vi "Escape String for JSON.vi"(11 "string":string) -> (3 "quoted string":string)   [LabVIEW 2020, in "Multi Error Cluster.lvlib"]
doc: "Convert reserved JSON characters into \\ escaped character sequences. This allows a name to contain a /, '\", \\, or a control character."
uses:
  <vilib>/MultiError/TokenizeJSON/Multi Error Cluster.lvlib
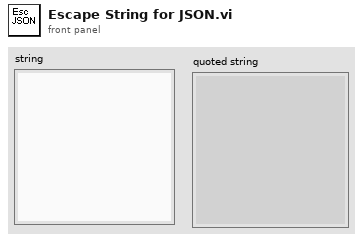
[diagram p1: front panel]
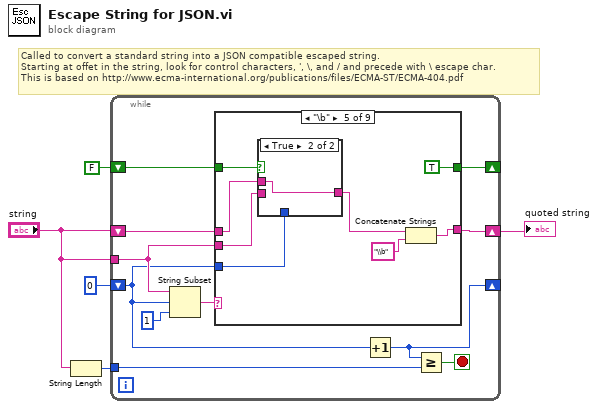
[diagram p0: block diagram]
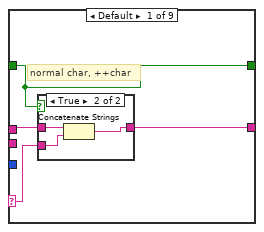
[diagram p2: hidden frame]
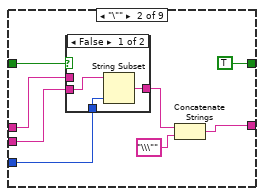
[diagram p4: hidden frame]
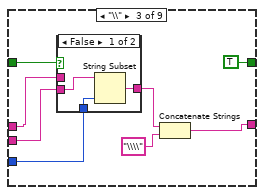
[diagram p6: hidden frame]
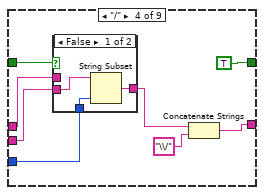
[diagram p8: hidden frame]
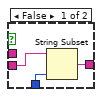
[diagram p10: hidden frame]
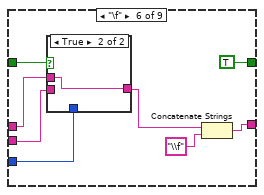
[diagram p11: hidden frame]
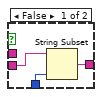
[diagram p12: hidden frame]
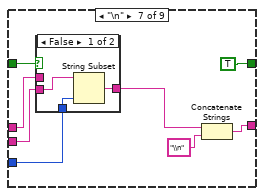
[diagram p13: hidden frame]
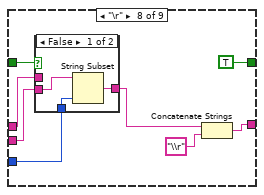
[diagram p15: hidden frame]
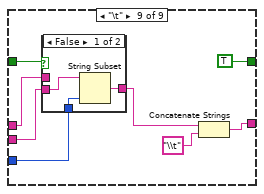
[diagram p17: hidden frame]
diagram:
  # "Called to convert a standard string into a JSON compatible escaped string.\nStarting at offet in the string, look for control characters, ', \\, and / and precede with \\ escape char.\nThis is based on http://www.ecma-international.org/publications/files/ECMA-ST/ECMA-404.pdf"
  n1 = String Length(string="string") -> (length=w5:i32)
  n2 = while {
    shift-right: [w10] -> w1
    shift-left: "string" -> [w11]
    shift-right: [w8] -> _
    shift-left: 0 ("offset") -> [w6]
    tunnel: w5 -> [w14]
    shift-right: [w9] -> _
    shift-left: FALSE -> [w12]
    tunnel: "string" -> [w7]
    stop <- w13 stop-if-true
    n3 = String Subset(string=w7, offset (0)=w6, length (rest)=1) -> (substring=w15:string)
    n4 = case shown="\"\\b\"" w15 {
      selector: w15 -> [w18 _ _ _ _ _ _ _ _]
      tunnel: w11 -> [w20 w28 w39 w52 w64 w77 w88 w100 w110]
      tunnel: w12 -> [w17 w29 w41 w53 w65 w75 w89 w101 w113]
      tunnel: [w19 w31 w43 w55 w67 w79 w91 w103 w115] -> w10
      tunnel: [w17 TRUE TRUE TRUE TRUE TRUE TRUE TRUE TRUE] -> w9
      tunnel: w7 -> [_ w27 w38 w51 w63 w76 w87 w99 w111]
      tunnel: w6 -> [_ w26 w37 w50 w62 w74 w86 w98 w112]
      frame Default {
        # "normal char, ++char"
        n5 = case shown="True" w17 {
          tunnel: w20 -> [w21 w24]
          tunnel: [w21 w22] -> w19
          tunnel: w18 -> [_ w23]
          frame False {
          }
          frame True {
            n6 = Concatenate Strings(w24, w23) -> (w22:string)
          }
        }
      }
      frame "\"" {
        n7 = case shown="False" w29 {
          tunnel: w28 -> [_ w36]
          tunnel: [w33 w36] -> w25
          tunnel: w27 -> [w35 _]
          tunnel: w26 -> [w34 _]
          frame False {
            n8 = String Subset(string=w35, length (rest)=w34) -> (substring=w33:string)  [unwired: 1 in]
          }
          frame True {
          }
        }
        n9 = Concatenate Strings(w25, "\\\"") -> (w31:string)
      }
      frame "\\" {
        n10 = case shown="False" w41 {
          tunnel: w39 -> [_ w48]
          tunnel: [w46 w48] -> w40
          tunnel: w37 -> [w47 _]
          tunnel: w38 -> [w45 _]
          frame False {
            n11 = String Subset(string=w45, length (rest)=w47) -> (substring=w46:string)  [unwired: 1 in]
          }
          frame True {
          }
        }
        n12 = Concatenate Strings(w40, "\\\\") -> (w43:string)
      }
      frame "/" {
        n13 = case shown="False" w53 {
          tunnel: w52 -> [_ w60]
          tunnel: [w57 w60] -> w49
          tunnel: w51 -> [w59 _]
          tunnel: w50 -> [w58 _]
          frame False {
            n14 = String Subset(string=w59, length (rest)=w58) -> (substring=w57:string)  [unwired: 1 in]
          }
          frame True {
          }
        }
        n15 = Concatenate Strings(w49, "\\/") -> (w55:string)
      }
      frame "\b" {
        n16 = case shown="True" w65 {
          tunnel: [w69 w72] -> w61
          tunnel: w63 -> [w71 _]
          tunnel: w62 -> [w70 _]
          tunnel: w64 -> [_ w72]
          frame False {
            n17 = String Subset(string=w71, length (rest)=w70) -> (substring=w69:string)  [unwired: 1 in]
          }
          frame True {
          }
        }
        n18 = Concatenate Strings(w61, "\\b") -> (w67:string)
      }
      frame "\f" {
        n19 = case shown="True" w75 {
          tunnel: [w81 w84] -> w73
          tunnel: w76 -> [w83 _]
          tunnel: w74 -> [w82 _]
          tunnel: w77 -> [_ w84]
          frame False {
            n20 = String Subset(string=w83, length (rest)=w82) -> (substring=w81:string)  [unwired: 1 in]
          }
          frame True {
          }
        }
        n21 = Concatenate Strings(w73, "\\f") -> (w79:string)
      }
      frame "\n" {
        n22 = case shown="False" w89 {
          tunnel: w88 -> [_ w96]
          tunnel: [w93 w96] -> w85
          tunnel: w87 -> [w95 _]
          tunnel: w86 -> [w94 _]
          frame False {
            n23 = String Subset(string=w95, length (rest)=w94) -> (substring=w93:string)  [unwired: 1 in]
          }
          frame True {
          }
        }
        n24 = Concatenate Strings(w85, "\\n") -> (w91:string)
      }
      frame "\r" {
        n25 = case shown="False" w101 {
          tunnel: w100 -> [_ w108]
          tunnel: [w105 w108] -> w97
          tunnel: w99 -> [w107 _]
          tunnel: w98 -> [w106 _]
          frame False {
            n26 = String Subset(string=w107, length (rest)=w106) -> (substring=w105:string)  [unwired: 1 in]
          }
          frame True {
          }
        }
        n27 = Concatenate Strings(w97, "\\r") -> (w103:string)
      }
      frame "\t" {
        n28 = case shown="False" w113 {
          tunnel: w110 -> [_ w120]
          tunnel: [w117 w120] -> w109
          tunnel: w111 -> [w119 _]
          tunnel: w112 -> [w118 _]
          frame False {
            n29 = String Subset(string=w119, length (rest)=w118) -> (substring=w117:string)  [unwired: 1 in]
          }
          frame True {
          }
        }
        n30 = Concatenate Strings(w109, "\\t") -> (w115:string)
      }
    }
    n31 = Increment(x=w6) -> (x+1=w8:i32)
    n32 = Greater Or Equal?(x=w8, y=w14) -> (x >= y?=w13:bool)
  }
  "quoted string" <- w1
